vi "XNET Frame to Signals List.vi"(8 "error in (no error)":errorcluster, 10 "XNET Frame":refnum<k21>, 11 "BS1200 in":refnum<class "BS120x.lvclass">) -> (0 "error out":errorcluster, 2 "Sorted XNET Signals":refnum<k21>[](array[refnum]), 3 "BS1200 out":refnum<class "BS120x.lvclass">)   [LabVIEW 2021, in "BS120x Driver.lvlib" / "BS120x.lvclass"]
uses:
  BS120x.lvclass
  BS120x.lvclass/BS120x.ctl
  <resource>/objmgr/xnet.rc
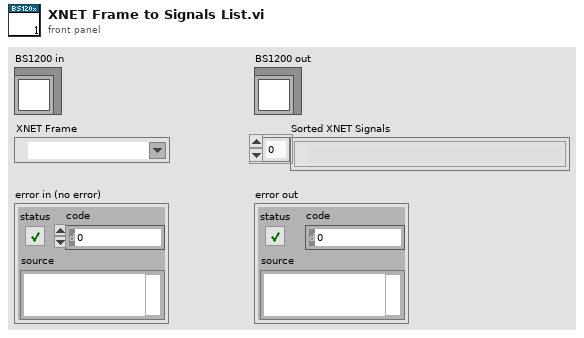
[diagram p1: front panel]
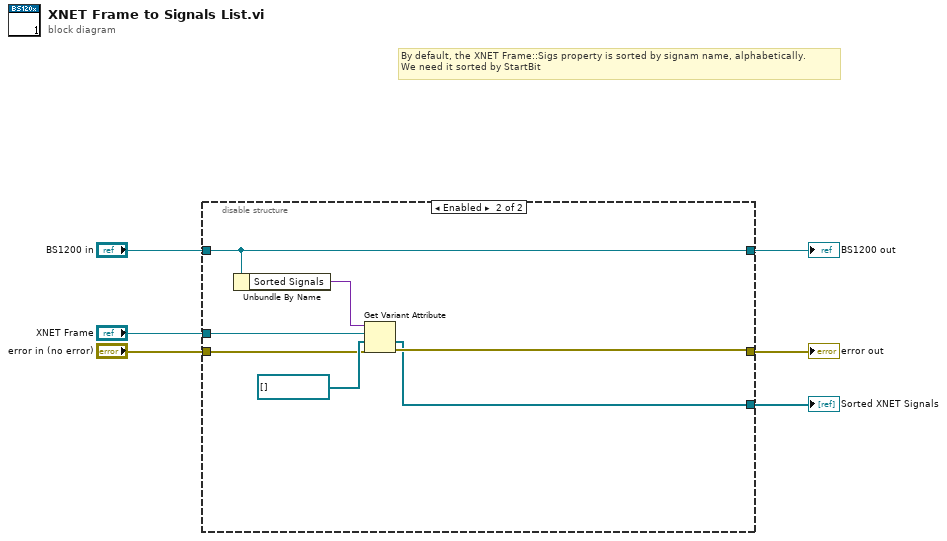
[diagram p0: block diagram]
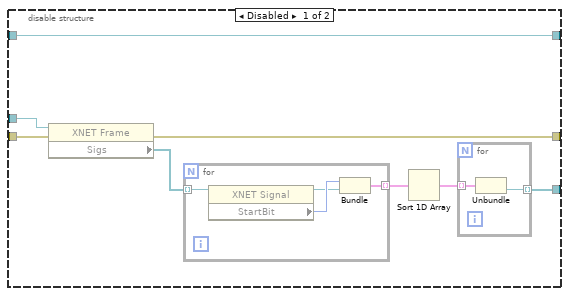
[diagram p2: hidden frame]
diagram:
  # "By default, the XNET Frame::Sigs property is sorted by signam name, alphabetically.\nWe need it sorted by StartBit"
  n1 = disable-structure shown="Enabled" {
    disable-tunnel: [w13 w21] -> w5
    disable-tunnel: "error in (no error)" -> [w12 w23]
    disable-tunnel: [w11 w22] -> w3
    disable-tunnel: "XNET Frame" -> [w10 w25]
    disable-tunnel: [w6 w20] -> _
    disable-tunnel: "BS1200 in" -> [w6 w20]
    frame Disabled {
      n2 = property class="XNET Frame"(reference=w10, error in=w12) -> (error out=w11:errorcluster, "Sigs"=w9:refnum<k21>[])  [unwired: 1 out]
      n3 = for {
        tunnel: w9 -> [w18] mode=indexing
        tunnel: [w16] -> w8 mode=indexing
        n4 = property class="XNET Signal"(reference=w18) -> (reference out=w17:refnum<k21>, "StartBit"=w19:u32)  [unwired: 1 in, 1 out]
        n5 = Bundle("StartBit"=w19, w17) -> (w16:cluster{"StartBit":u32, refnum<k21>})  [unwired: 1 in]
      }
      n6 = Sort 1D Array(array=w8) -> (sorted array=w7:cluster{"StartBit":u32, refnum<k21>}[])
      n7 = for {
        tunnel: w7 -> [w15] mode=indexing
        tunnel: [w14] -> w13 mode=indexing
        n8 = Unbundle(w15) -> (w14:refnum<k21>)  [unwired: 1 out]
      }
    }
    frame Enabled {
      n9 = Unbundle By Name(w20) -> ("Sorted Signals"=w26:variant)
      n10 = Get Variant Attribute(Variant=w26, name=w25, default value (empty Variant)=refnum<k21>[] [] ("Sorted XNET Signals"), error in=w23) -> (value=w21:refnum<k21>[], error out=w22:errorcluster)  [unwired: 2 out]
    }
  }
  "Sorted XNET Signals" <- w5
  "error out" <- w3
  "BS1200 out" <- "BS1200 in"
